vi "ctx set sensor compensation data.vi"(9 "sensor_index":i32, 10 "src_comp_data":T1, 11 "context":u32) -> (2 "function return":i32, 3 "context out":u32)   [LabVIEW 2019, in "apdm.lvlib"]
doc: "APDM_EXPORT int apdm_ctx_set_sensor_compensation_data(apdm_ctx_t context, const apdm_sensor_compensation_t *src_comp_data, const int32_t sensor_index);"
uses:
  apdm.lvlib
  Lee Lab/CP FES Walking 2018/Code/Working/LabVIEW/apdm.dll
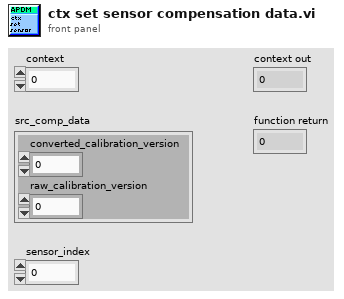
[diagram p1: front panel]
types:
  T1 = cluster{"converted_calibration_version":u32, "raw_calibration_version":u32}
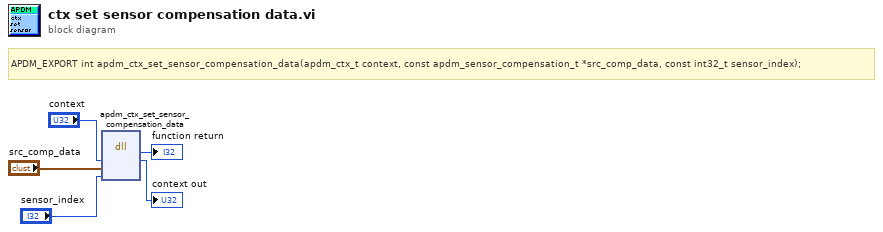
[diagram p0: block diagram]
diagram:
  # "APDM_EXPORT int apdm_ctx_set_sensor_compensation_data(apdm_ctx_t context, const apdm_sensor_compensation_t *src_comp_data, const int32_t sensor_index);"
  n1 = dll-call lib="C:/Users/jfalesi/Dropbox/Lee Lab/CP FES Walking 2018/Code/Working/LabVIEW/apdm.*" fn="apdm_ctx_set_sensor_compensation_data"("context"="context", "src_comp_data"="src_comp_data", "sensor_index"="sensor_index") -> (→"function return":i32, "context"=→"context out":u32)  [unwired: 5 in, 2 out]
